vi "write_ht3_header_file.vi"(5 "Data_path":path, 6 "sync_rate":i32, 8 "error in (no error)":errorcluster, 9 "Notes":string, 11 "swabian_local_data in":T1={"events"={"update_status"=refnum, "update_chart"=refnum, "update_xy"=refnum, "send_channel_data"=refnum}, "stop_q"=refnum, "tagger_reference"=refnum, "connect_button"=refnum, "counter_reference"=refnum, "tagger_stream_reference"=refnum, "log_reference"=refnum, "current_log_offset"=0, "tt20_buffer_q"=refnum, "stream_to_file_button"=refnum, "num_records"=0, "connected?"=FALSE, "plots"=refnum, "histogram_bin_edges"=[], "histogrammer"=refnum, "plot_lifetimes"=refnum, "xy_graph"=refnum, "Reference\nChannel"=enum."ch0", "trigger_channels"=[], "filter_channels"=[], "active_channels"=[], "acq_mode"=0, "Reference\nChannel"=enum."ch0", "acq_time"=0, "first_batch?"=FALSE, "first_sync_stamp"=0, "leftovers"={"leftover_stamps"=[], "leftover_channels"=[], "any?"=FALSE}}) -> (0 "error out":errorcluster, 3 "swabian_local_data in 2":T1={"events"={"update_status"=refnum, "update_chart"=refnum, "update_xy"=refnum, "send_channel_data"=refnum}, "stop_q"=refnum, "tagger_reference"=refnum, "connect_button"=refnum, "counter_reference"=refnum, "tagger_stream_reference"=refnum, "log_reference"=refnum, "current_log_offset"=0, "tt20_buffer_q"=refnum, "stream_to_file_button"=refnum, "num_records"=0, "connected?"=FALSE, "plots"=refnum, "histogram_bin_edges"=[], "histogrammer"=refnum, "plot_lifetimes"=refnum, "xy_graph"=refnum, "Reference\nChannel"=enum."ch0", "trigger_channels"=[], "filter_channels"=[], "active_channels"=[], "acq_mode"=0, "Reference\nChannel"=enum."ch0", "acq_time"=0, "first_batch?"=FALSE, "first_sync_stamp"=0, "leftovers"={"leftover_stamps"=[], "leftover_channels"=[], "any?"=FALSE}})   [LabVIEW 2018]
uses:
  swabian_local_data_tdef.ctl
  swabian_events_tdef.ctl
  update_chart_tdef.ctl
  channel_data_tdef.ctl
  C:/Users/SWIR TCSPC/Desktop/Swabian/lib/TTCSharp32.dll
  lib/TTCSharp32.dll
  swabian_buffer_tdef.ctl
  reference_checkbox_tdef.ctl
  leftovers_struct.ctl
panel:
  out "concatenated string":string
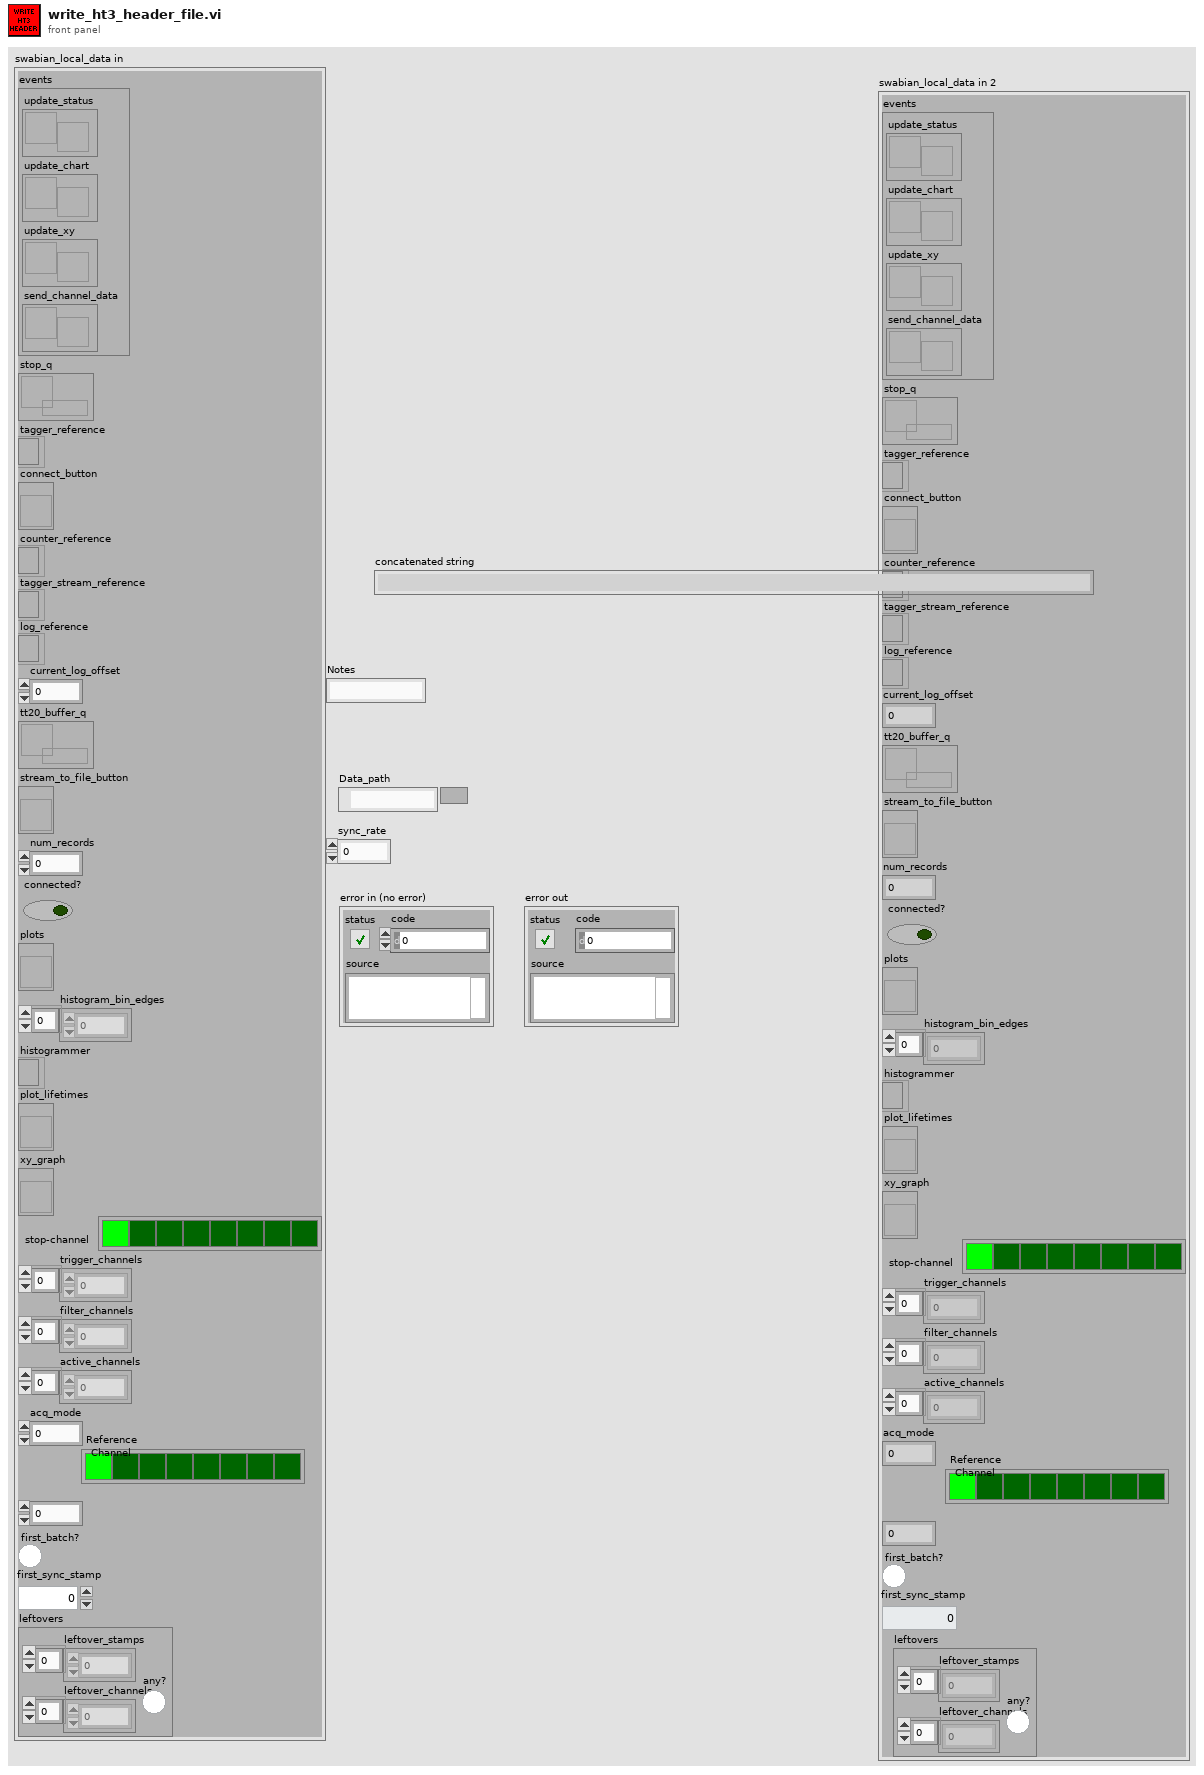
[diagram p1: front panel]
types:
  T1 = typedef "swabian_local_data_tdef.ctl" = cluster{"events":T2, "stop_q":refnum<queue>, "tagger_reference":refnum<k24>, "connect_button":refnum<vi>, "counter_reference":refnum<k24>, "tagger_stream_reference":refnum<k24>, "log_reference":refnum<file>, "current_log_offset":i64, "tt20_buffer_q":refnum<queue>, "stream_to_file_button":refnum<vi>, "num_records":u64, "connected?":bool, "plots":refnum<vi>, "histogram_bin_edges":i64[], "histogrammer":refnum<k24>, "plot_lifetimes":refnum<vi>, "xy_graph":refnum<vi>, "Reference\nChannel":T3, "trigger_channels":i32[], "filter_channels":i32[], "active_channels":i32[], "acq_mode":i32, "Reference\nChannel":T3, "acq_time":i64, "first_batch?":bool, "first_sync_stamp":i64, "leftovers":T4}
  T2 = typedef "swabian_events_tdef.ctl" = cluster{"update_status":refnum<user-event>, "update_chart":refnum<user-event>, "update_xy":refnum<user-event>, "send_channel_data":refnum<user-event>}
  T3 = typedef "reference_checkbox_tdef.ctl" = enum32{"No Selection", "ch0", "ch1", "ch2", "ch3", "ch4", "ch5", "ch6", "ch7"}
  T4 = typedef "leftovers_struct.ctl" = cluster{"leftover_stamps":i64[], "leftover_channels":i32[], "any?":bool}
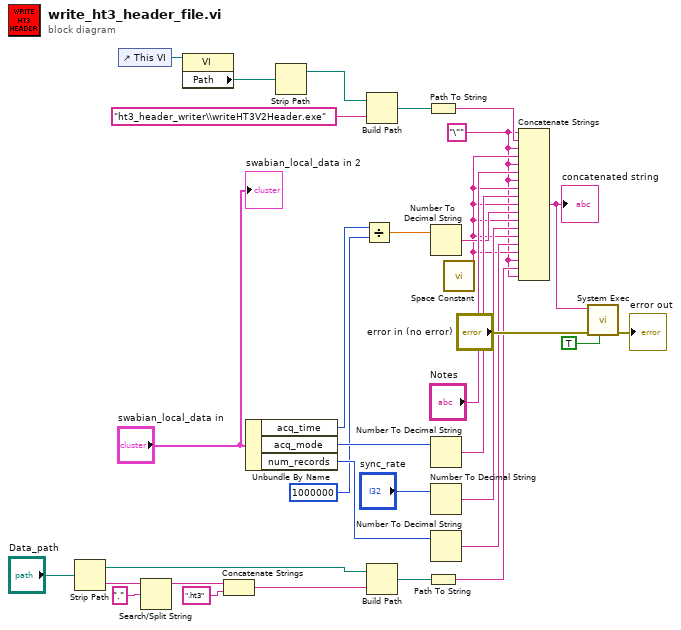
[diagram p0: block diagram]
diagram:
  w6 = "\""
  n1 = Strip Path(path="Data_path") -> (stripped path=w26:path, name=w28:string)
  n2 = control-ref of="This VI"() -> (w24:refnum<vi>)
  n3 = Search/Split String(string=w28, search string/char (-)="." ("regular expression")) -> (substring before match=w30:string)  [unwired: 1 in, 2 out]
  n4 = property class="VI"(reference=w24) -> ("Path"=w23:path)  [unwired: 1 in, 2 out]
  n5 = Concatenate Strings(w30, ".ht3" ("string")) -> (w32:string)
  n6 = Unbundle By Name("swabian_local_data in") -> ("acq_time"=w3:i64, "acq_mode"=w4:i32, "num_records"=w11:u64)
  n7 = Strip Path(path=w23) -> (stripped path=w22:path)  [unwired: 1 out]
  n8 = Divide(x=w3, y=i64 1000000) -> (x/y=w1:dbl)
  n9 = Build Path(base path=w22, name or relative path="ht3_header_writer\\writeHT3V2Header.exe") -> (appended path=w21:path)
  n10 = Build Path(base path=w26, name or relative path=w32) -> (appended path=w8:path)
  n11 = Path To String(path=w21) -> (string=w18:string)
  n12 = Path To String(path=w8) -> (string=w7:string)
  n13 = Number To Decimal String(number=w1) -> (decimal integer string=w14:string)  [unwired: 1 in]
  n14 = Number To Decimal String(number=w4) -> (decimal integer string=w15:string)  [unwired: 1 in]
  n15 = Number To Decimal String(number="sync_rate") -> (decimal integer string=w12:string)  [unwired: 1 in]
  n16 = Number To Decimal String(number=w11) -> (decimal integer string=w10:string)  [unwired: 1 in]
  n17 = call <vilib>:"Space Constant.vi"() -> ("String"=w9:string)
  n18 = Concatenate Strings(w6, w18, w6, w9, w6, "Notes", w6, w9, w15, w9, w14, w9, w12, w9, w10, w9, w6, w7, w6) -> (w16:string)
  "concatenated string" <- w16
  n19 = call <vilib>:"System Exec.vi"("run minimized? (F)"=TRUE, "error in (no error)"="error in (no error)", "command line"=w16) -> ("error out"=→"error out":errorcluster)  [unwired: 5 in, 3 out]
  "swabian_local_data in 2" <- "swabian_local_data in"
